vi "uPolicy_TopicIsRelevant.vi"(8 "error in (no error)":errorcluster, 10 "Observed Topic (Lower Case)":string, 11 "Null in":refnum<class "Null.lvclass">) -> (0 "error out":errorcluster, 2 "Relevant?":bool, 3 "Null out":refnum<class "Null.lvclass">)   [LabVIEW 2023, in "uFramework_pack_uPolicy.lvlib" / "Null.lvclass"]
uses:
  Null.lvclass
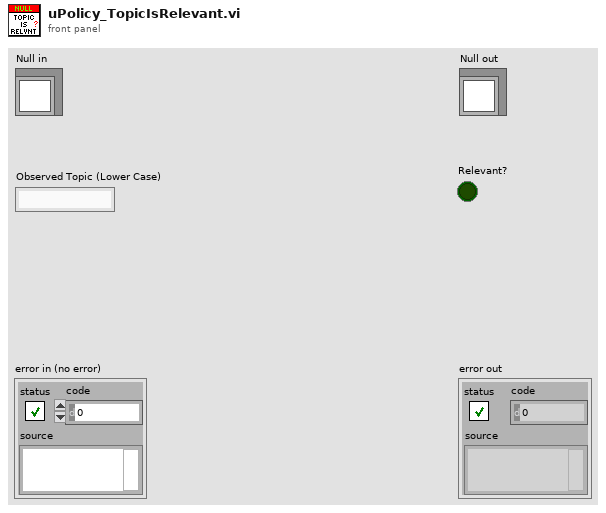
[diagram p1: front panel]
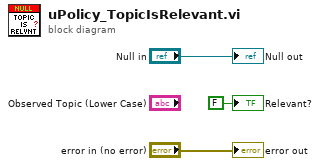
[diagram p0: block diagram]
diagram:
  "error out" <- "error in (no error)"
  "Null out" <- "Null in"
  "Relevant?" <- FALSE ("Relevant?")
